vi "Main ver4.vi"(0 "PID On":bool) -> (5 "Total (V)":dbl[](array[slide]) scale=-8.0..8.0, 6 "Force (N)":T1(graph)={"M1 ref force"=19.690402476780186, "M2 ref force"=19.690402476780186, "M1 mes force"=5.466389475814116, "M2 mes force"=1.4423805363163493})   [LabVIEW 2021]
uses:
  <vilib>/Platform/TimedLoop/XDataNode/timing_clust.ctl
  <vilib>/Platform/TimedLoop/XDataNode/nitl_modes.ctl
  <vilib>/Platform/TimedLoop/XDataNode/wakeup.ctl
  <vilib>/Analysis/3filter.llb/Filter Passband Type.ctl
  <vilib>/Analysis/baseanly.llb/Real Dot Product.vi
  <vilib>/DAQmx/write.llb/DAQmx Write (Digital 1D Bool 1Chan 1Samp).vi
  <vilib>/DAQmx/write.llb/DAQmx Write (Analog 1D DBL NChan 1Samp).vi
  <vilib>/DAQmx/create/channels.llb/DAQmx Create Channel (DO-Digital Output).vi
  <vilib>/DAQmx/create/channels.llb/DAQmx Create Channel (AO-Voltage-Basic).vi
  <vilib>/DAQmx/create/channels.llb/DAQmx Create Channel (AI-Voltage-Basic).vi
  <vilib>/DAQmx/configure/timing.llb/DAQmx Timing (Sample Clock).vi
  <vilib>/addons/control/pid/pid.llb/PID (DBL).vi
  <vilib>/DAQmx/miscellaneous.llb/DAQmx Fill In Error Info.vi
  <vilib>/platform/TimedLoop/XDataNode/XDataNode.xnode
  <vilib>/addons/control/pid/NI_PID_pid.lvlib
  <vilib>/Platform/TimedLoop/XDataNode/XDNodeRunTimeDep.lvlib
  <vilib>/Analysis/NI_AALBase.lvlib
  <vilib>/ptbypt/NI_PtbyPt.lvlib
panel:
  out "Force (N) 2":T1(graph)={"M1 ref force"=19.938080495356036, "M2 ref force"=19.938080495356036, "M1 mes force"=7.2507342741854055, "M2 mes force"=-127.25356072908707}
  in  "Gains 2":T2(array[cluster])=[{"proportional gain (Kc)"=0.17, "integral time (Ti, min)"=0.0, "derivative time (Td, min)"=0.0}, {"proportional gain (Kc)"=0.17, "integral time (Ti, min)"=0.0, "derivative time (Td, min)"=0.0}] {"derivative time (Td, min)" format="%.3f"; "integral time (Ti, min)" format="%.3f"; "proportional gain (Kc)" format="%.3f"}
  in  "Torque":dbl[](array[numeric])=[0.15, 0.15]
  out "Speed":dbl[](array[numeric])
  in  "Record?":bool
  out "XY Graph":cluster{dbl[], dbl[]}[](graph)=[{[0.0, 26.31578947368421, 52.63157894736842, 78.94736842105263, 105.26315789473684, 131.57894736842104, 157.89473684210526, 184.21052631578945, 210.52631578947367, 236.8421052631579, 263.1578947368421, 289.4736842105263, 315.7894736842105, 342.10526315789474, 368.4210526315789, 394.7368421052631, 421.05263157894734, 447.36842105263156, 473.6842105263158, 499.99999999999994], [0.0, 0.0, 0.0, 0.0, 0.0, 0.0, 0.0, 0.0, 0.0, 0.0, 0.0, 0.0, 0.0, 0.0, 0.0, 0.0, 0.0, 0.0, 0.0, 0.0]}, {[0.0, 26.31578947368421, 52.63157894736842, 78.94736842105263, 105.26315789473684, 131.57894736842104, 157.89473684210526, 184.21052631578945, 210.52631578947367, 236.8421052631579, 263.1578947368421, 289.4736842105263, 315.7894736842105, 342.10526315789474, 368.4210526315789, 394.7368421052631, 421.05263157894734, 447.36842105263156, 473.6842105263158, 499.99999999999994], [0.0, 0.0, 0.0, 0.0, 0.0, 0.0, 0.0, 0.0, 0.0, 0.0, 0.0, 0.0, 0.0, 0.0, 0.0, 0.0, 0.0, 0.0, 0.0, 0.0]}, {[0.0, 26.31578947368421, 52.63157894736842, 78.94736842105263, 105.26315789473684, 131.57894736842104, 157.89473684210526, 184.21052631578945, 210.52631578947367, 236.8421052631579, 263.1578947368421, 289.4736842105263, 315.7894736842105, 342.10526315789474, 368.4210526315789, 394.7368421052631, 421.05263157894734, 447.36842105263156, 473.6842105263158, 499.99999999999994], [0.0, 0.0, 0.0, 0.0, 0.0, 0.0, 0.0, 0.0, 0.0, 0.0, 0.0, 0.0, 0.0, 0.0, 0.0, 0.0, 0.0, 0.0, 0.0, 0.0]}, {[0.0, 26.31578947368421, 52.63157894736842, 78.94736842105263, 105.26315789473684, 131.57894736842104, 157.89473684210526, 184.21052631578945, 210.52631578947367, 236.8421052631579, 263.1578947368421, 289.4736842105263, 315.7894736842105, 342.10526315789474, 368.4210526315789, 394.7368421052631, 421.05263157894734, 447.36842105263156, 473.6842105263158, 499.99999999999994], [0.0, 0.0, 0.0, 0.0, 0.0, 0.0, 0.0, 0.0, 0.0, 0.0, 0.0, 0.0, 0.0, 0.0, 0.0, 0.0, 0.0, 0.0, 0.0, 0.0]}]
  out "Period":i64=2
  out "Finished Late? [i-1]":bool
  in  "Tab Control 2":enum32{"Initialize", "RBF"}(tab)
  in  "Encoder":bool
  in  "Loadcell":bool
  in  "Set Tension":dbl=10.0
  in  "x":cluster{"Number":i32, "x_0":dbl, "x_f":dbl}={"Number"=20, "x_0"=0.0, "x_f"=500.0}
  out "Output":dbl(slide)=nan scale=0.0..10.0
  out "Weights":dbl[](array[numeric])
  in  "RBF 2":cluster{"STD":dbl, "Number":i32}={"STD"=150.0, "Number"=3}
  in  "Traj Start":i32(knob)=1 scale=0.0..2.0
  in  "Tab Control":enum32{"Page 1", "Position"}(tab)=enum."Position"
  out "RPM":cluster{"Position":dbl, "ref_x (mm)":dbl}(graph)
  out "Position (mm)":cluster{"Position":dbl, "ref_x (mm)":dbl}(graph)={"Position"=0.0, "ref_x (mm)"=500.0}
  in  "RBF":bool
  in  "Set Point":dbl(slide)=19.938080495356036 scale=0.0..40.0
  in  "stop":bool
  in  "Tab Control 3":enum32{"Current", "PID On", "Position"}(tab)=enum."PID On"
  in  "Gains":T2(array[cluster])=[{"proportional gain (Kc)"=0.17, "integral time (Ti, min)"=0.0, "derivative time (Td, min)"=0.0}, {"proportional gain (Kc)"=0.17, "integral time (Ti, min)"=0.0, "derivative time (Td, min)"=0.0}] {"derivative time (Td, min)" format="%.3f"; "integral time (Ti, min)" format="%.3f"; "proportional gain (Kc)" format="%.3f"}
  out "PID (V)":dbl[](array[slide])=[2.9907120743034055, 2.9907120743034055] scale=-8.0..10.0
  in  "Motor Enable":bool[](array[boolean])=[FALSE, FALSE]
  in  "Damping":dbl[](array[numeric])=[0.0, 0.0]
  in  "PID gains":T3={"proportional gain (Kc)"=0.1, "integral time (Ti, min)"=0.0, "derivative time (Td, min)"=0.0} {"derivative time (Td, min)" format="%.3f"; "integral time (Ti, min)" format="%.3f"; "proportional gain (Kc)" format="%.3f"}
  in  "Pos Control":bool
  out "output":dbl(slide)=50.0 scale=-40.0..40.0
  # "TRAJECTORY"
  # "FORCE"
  # "INITIALIZE"
  # "TUNE"
  # "MONITOR"
  # "DEVEL"
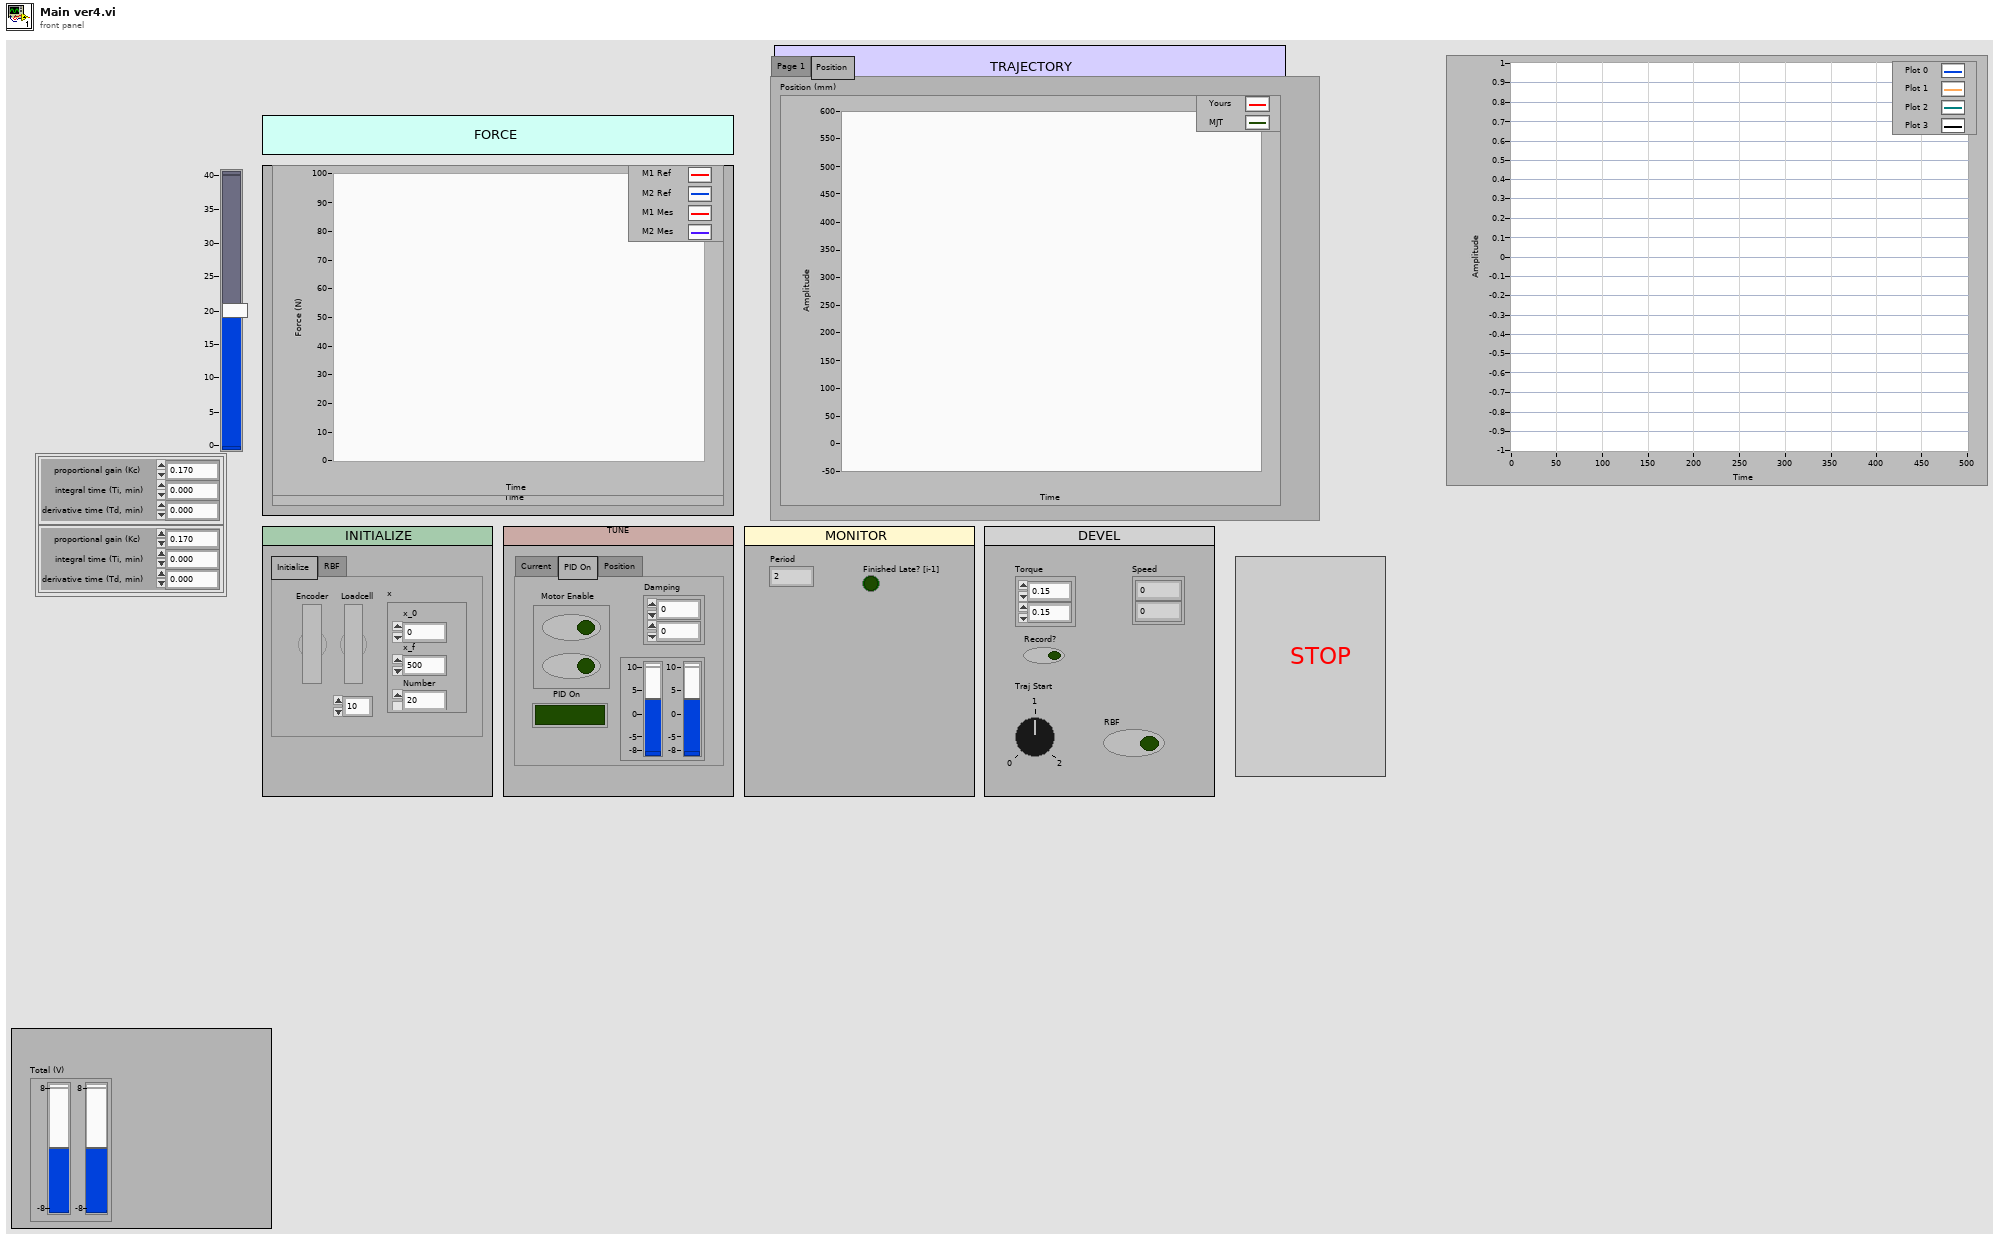
[diagram p1: front panel]
types:
  T1 = cluster{"M1 ref force":dbl, "M2 ref force":dbl, "M1 mes force":dbl, "M2 mes force":dbl}
  T2 = cluster{"proportional gain (Kc)":dbl, "integral time (Ti, min)":dbl, "derivative time (Td, min)":dbl}[]
  T3 = cluster{"proportional gain (Kc)":dbl, "integral time (Ti, min)":dbl, "derivative time (Td, min)":dbl}
  T4 = enum16{"open", "open or create", "create or replace", "create", "open (read-only)"}
  T5 = typedef "XDNodeRunTimeDep.lvlib/timing_clust.ctl" = cluster{"Expected End [f-1]":u64, "Actual End [f-1]":u64, "Finished Late? [f-1]":bool, "Expected End [i-1]":u64, "Actual End [i-1]":u64, "Finished Late? [i-1]":bool, "Expected Start [i]":u64, "Actual Start [i]":u64, "Expected Start [f]":u64, "Actual Start [f]":u64, "Source Name":string, "Structure Name":string, "Period":i64, "Deadline":i64, "Offset":i64, "Start":i64, "Priority":i32, "Timeout":i32, "Mode":T6, "Wakeup Reason":T7, "Error":errorcluster, "Source Type":string, "Secondary Source Type":string, "Global End Time":u64, "Global Start Time":u64, "Frame Duration":u64, "Iteration Duration":u64, "Assigned CPU":i32, "I/O Scan Engine Mode":u32}
  T6 = typedef "XDNodeRunTimeDep.lvlib/nitl_modes.ctl" = enum32{"No Change", "Process missed periods, maintain original phase", "Discard missed periods, maintain original phase", "Process missed periods, ignore original phase", "Discard missed periods, ignore original phase"}
  T7 = typedef "XDNodeRunTimeDep.lvlib/wakeup.ctl" = enum32{"Normal", "Aborted", "Asynchronous wakeup", "Timing source error", "Timed loop error", "Timeout"}
  T8 = typedef "NI_AALBase.lvlib/Filter Passband Type.ctl" = enum32{"Lowpass", "Highpass", "Bandpass", "Bandstop"}
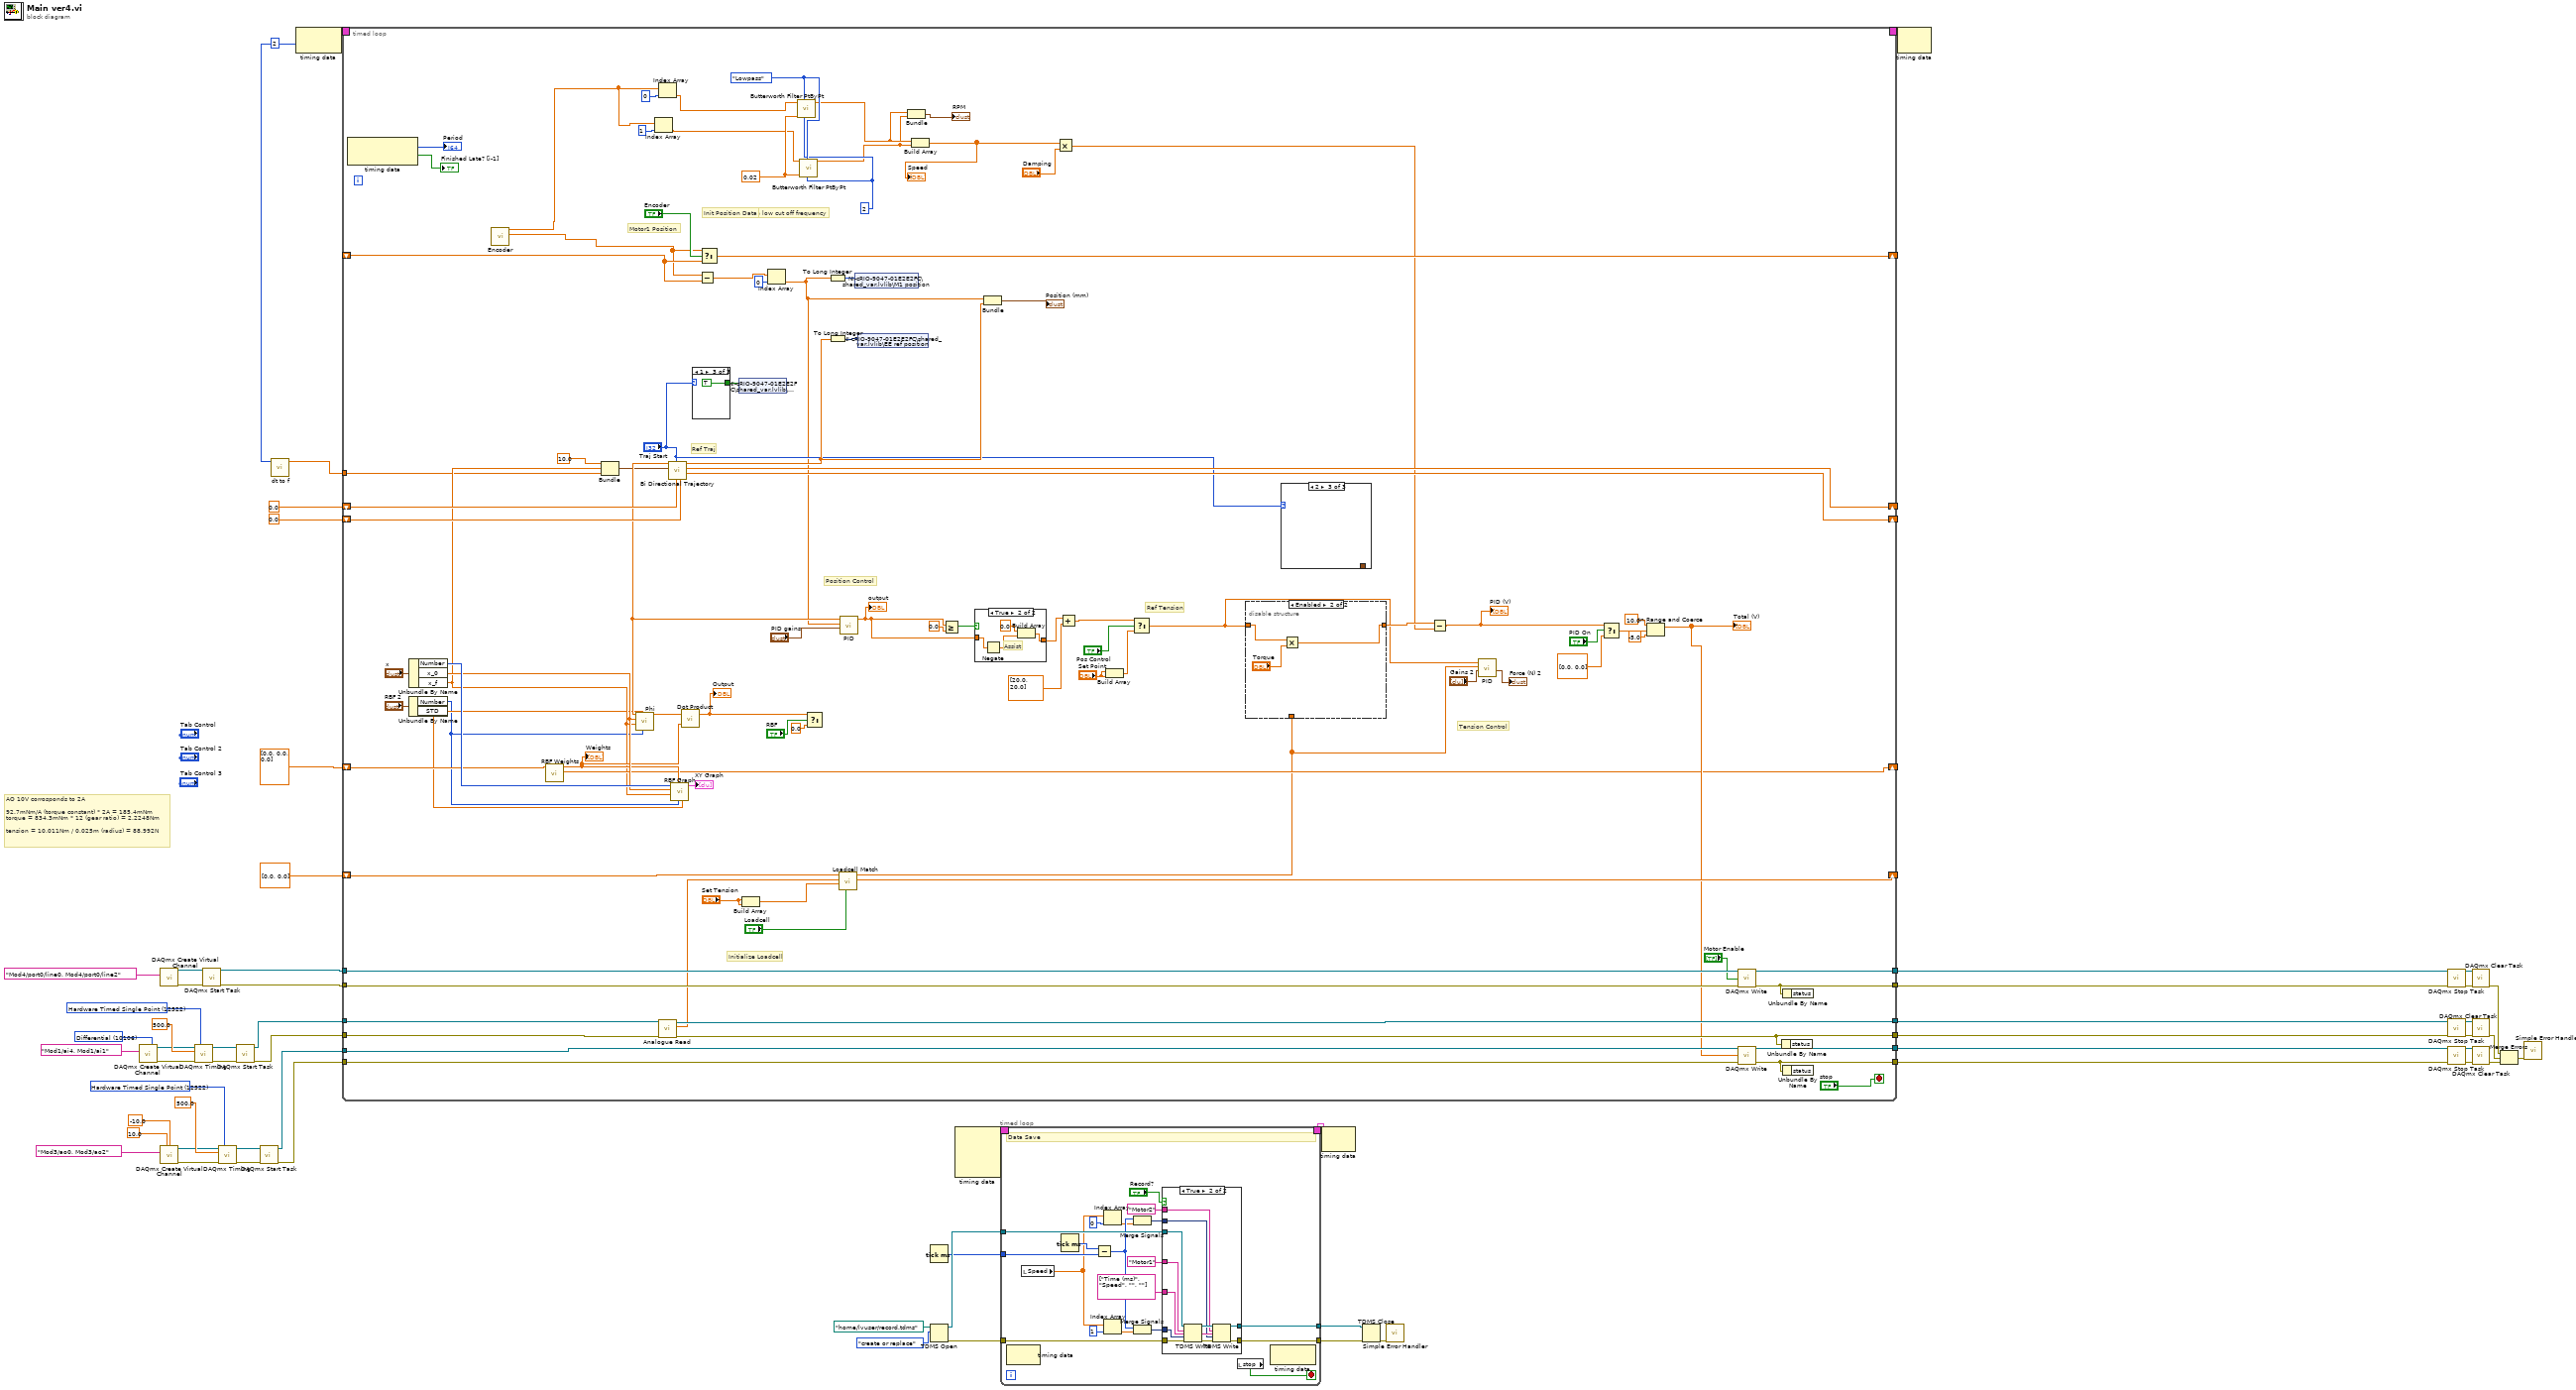
[diagram p0: block diagram]
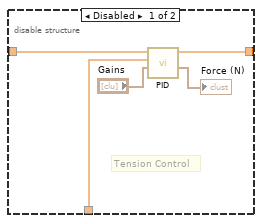
[diagram p3: hidden frame]
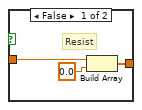
[diagram p4: hidden frame]
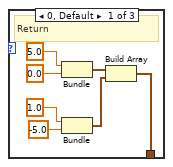
[diagram p5: hidden frame]
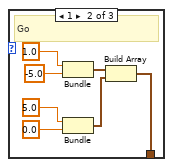
[diagram p6: hidden frame]
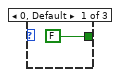
[diagram p7: hidden frame]
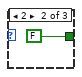
[diagram p8: hidden frame]
diagram:
  w15 = 12522 items=["Finite Samples"=10178, "Continuous Samples"=10123, "Hardware Timed Single Point"=12522] ("sample mode")
  w18 = 12522 items=["Finite Samples"=10178, "Continuous Samples"=10123, "Hardware Timed Single Point"=12522] ("sample mode")
  w25 = i64 2 ("Period")
  w32 = 10106 items=["Default"=-1, "RSE"=10083, "NRSE"=10078, "Differential"=10106, "Pseudodifferential"=12529] ("input terminal configuration")
  # "AO 10V corrosponds to 2A\n\n92.7mNm/A (torque constant) * 2A = 185.4mNm\ntorque = 834.3mNm * 12 (gear ratio) = 2.2248Nm\n\ntension = 10.011Nm / 0.025m (radius) = 88.992N"
  n1 = call-poly <vilib>:"DAQmx Create Virtual Channel.vi"("input terminal configuration"=w32, "physical channels"=tag "Mod1/ai4, Mod1/ai1") -> ("task out"=w22:refnum<k21>, "error out"=w21:errorcluster)  [unwired: 12 in]
  n2 = call-poly <vilib>:"DAQmx Create Virtual Channel.vi"("lines"=tag "Mod4/port0/line0, Mod4/port0/line2") -> ("task out"=w17:refnum<k21>, "error out"=w54:errorcluster)  [unwired: 13 in]
  n3 = call-poly <vilib>:"DAQmx Create Virtual Channel.vi"("maximum value"=10.0 ("AO max"), "minimum value"=-10.0 ("AO min"), "physical channels"=tag "Mod3/ao0, Mod3/ao2" ("Physical Channel(s)")) -> ("task out"=w14:refnum<k21>, "error out"=w12:errorcluster)  [unwired: 11 in]
  n4 = call-poly <vilib>:"DAQmx Timing.vi"("task/channels in"=w22, "sample mode"=w18, "rate"=500.0, "error in"=w21) -> ("task out"=w19:refnum<k21>, "error out"=w20:errorcluster)  [unwired: 10 in]
  n5 = call <vilib>:"DAQmx Start Task.vi"("task/channels in"=w17, "error in"=w54) -> ("task out"=w52:refnum<k21>, "error out"=w51:errorcluster)  [unwired: 12 in]
  n6 = call-poly <vilib>:"DAQmx Timing.vi"("task/channels in"=w14, "sample mode"=w15, "rate"=500.0, "error in"=w12) -> ("task out"=w13:refnum<k21>, "error out"=w11:errorcluster)  [unwired: 10 in]
  n7 = call <vilib>:"DAQmx Start Task.vi"("task/channels in"=w19, "error in"=w20) -> ("task out"=w45:refnum<k21>, "error out"=w44:errorcluster)  [unwired: 12 in]
  n8 = call <vilib>:"DAQmx Start Task.vi"("task/channels in"=w13, "error in"=w11) -> ("task out"=w56:refnum<k21>, "error out"=w55:errorcluster)  [unwired: 12 in]
  n9 = call "dt to f.vi"("Period"=w25) -> ("Frequency"=w24:dbl)  [unwired: 10 in]
  n10 = node-c288(w25) -> (w28:T5)
  n11 = timed-loop {
    tunnel: [w153] -> w60
    tunnel: [w152] -> w59
    tunnel: [w139] -> w58
    tunnel: [w144] -> w57
    tunnel: w45 -> [w150]
    tunnel: w44 -> [w149]
    tunnel: w56 -> [w138]
    tunnel: w55 -> [w151]
    tunnel: w52 -> [w148]
    tunnel: w51 -> [w147]
    tunnel: [w146] -> w48
    tunnel: [w145] -> w47
    shift-right: [w142] -> _
    shift-left: 0.0 ("total time") -> [w143]
    shift-right: [w141] -> _
    shift-left: _ -> [w140]
    shift-right: [w136] -> _
    shift-left: dbl[] [0.0, 0.0] ("measured force") -> [w137]
    shift-right: [w134] -> _
    shift-left: 0.0 ("total time") -> [w135]
    timing: w28 -> [_]
    timing-out: [_] -> w27
    shift-right: [w101] -> _
    shift-left: dbl[] [0.0, 0.0, 0.0] ("Array of Double") -> [w102]
    tunnel: w24 -> [w93]
    stop <- "stop" stop-if-true
    w83 = 2 ("order")
    w85 = 0.02 ("low cutoff freq: fl")
    w84 = Filter_Passband_Type."Lowpass" ("filter type")
    # "Tension Control"
    # "change low cut off frequency"
    # "Initialize Loadcell"
    # "Ref Tension"
    # "Position Control"
    # "Ref Traj"
    # "Init Position Data"
    # "Motor1 Position"
    n12 = node-c288() -> (→"Period":i64, →"Finished Late? [i-1]":bool)  [unwired: 1 in]
    n13 = Unbundle By Name("RBF 2") -> ("Number"=w89:i32, "STD"=w90:dbl)
    n14 = Unbundle By Name("x") -> ("Number"=w111:i32, "x_0"=w108:dbl, "x_f"=w94:dbl)
    n15 = call "Encoder.vi"() -> ("Mes Pos (mm)"=w72:dbl[], "RPM"=w80:dbl[])  [unwired: 10 in]
    n16 = call "RBF Weights.vi"("Array of Double in"=w102) -> ("Array of Double out"=w101:dbl[], "Array of Double 3"=w103:dbl[])  [unwired: 9 in]
    "Weights" <- w103
    n17 = Bundle("y"=10.0, "x_f"=w94, "Frequency"=w93) -> (w92:cluster{"y":dbl, "x_f":dbl, "Frequency":dbl})  [unwired: 1 in]
    n18 = Index Array(array=w80, index=1) -> (element=w78:dbl)
    n19 = Index Array(array=w80, index=0) -> (element=w79:dbl)
    n20 = call "Analogue Read.vi"("error in"=w149, "task/channels in"=w150) -> ("error out"=w144:errorcluster, "measured force"=w120:dbl[], "task out"=w139:refnum<k21>)  [unwired: 6 in, 1 out]
    n21 = call "Bi Directional Trajectory.vi"("Return Time"=w135, "Go Time"=w143, "Traj Start"="Traj Start", "Trajectory Settings"=w92) -> ("Return Next Time"=w134:dbl, "Go Next Time"=w142:dbl, "Output (mm)"=w107:dbl)  [unwired: 5 in]
    n22 = call "Phi.vi"("Number"=w89, "STD"=w90, "x_f"=w94, "x_0"=w108, "Output (mm)"=w107) -> ("Array"=w106:dbl[])  [unwired: 6 in]
    n23 = call "RBF Graph.vi"("STD"=w90, "Number"=w89, "Array of Double 3"=w103, "x_f"=w94, "x_0"=w108, "Number 2"=w111) -> ("Array"=→"XY Graph":cluster{dbl[], dbl[]}[])  [unwired: 5 in]
    n24 = call-poly <vilib>:"Dot Product.vi"("Y Vector"=w103, "X Vector"=w106) -> ("X * Y"=w100:dbl)  [unwired: 1 out]
    "Output" <- w100
    n25 = case shown="1" "Traj Start" {
      tunnel: [FALSE FALSE TRUE] -> w104
      frame 0, Default {
      }
      frame 2 {
      }
      frame 1 {
      }
    }
    n26 = Subtract(x=w72, y=w140) -> (x-y=w71:dbl[])
    n27 = Select(t=w72, s="Encoder", f=w140) -> (s? t:f=w141:dbl[])
    n28 = shared-variable "NI-cRIO-9047-01E2E2FC\\shared_var.lvlib\\Trigger"(w104) -> ()  [unwired: 1 in, 1 out]
    n29 = Build Array("Set Tension", "Set Tension") -> (w118:dbl[])
    n30 = Index Array(array=w71, index=0) -> (element=w70:dbl)
    n31 = call <vilib>:"Butterworth Filter PtByPt.vi"("order"=w83, "filter type"=w84, "low cutoff freq: fl"=w85, "x"=w79) -> ("Filtered x"=w68:dbl)  [unwired: 5 in, 1 out]
    n32 = call <vilib>:"Butterworth Filter PtByPt.vi"("order"=w83, "filter type"=w84, "low cutoff freq: fl"=w85, "x"=w78) -> ("Filtered x"=w67:dbl)  [unwired: 5 in, 1 out]
    n33 = Select(t=w100, s="RBF", f=0.0) -> ()  [unwired: 1 out]
    n34 = To Long Integer(number=w70) -> (32bit integer=w114:i32)
    n35 = To Long Integer(number=w107) -> (32bit integer=w115:i32)
    n36 = call "Loadcell Match.vi"("Initialize"="Loadcell", "Set Tension"=w118, "Mes Tension"=w120, "Next Tension Error"=w137) -> ("Tension Error"=w136:dbl[], "Filtered Tension"=w61:dbl[])  [unwired: 6 in]
    n37 = call-poly <vilib>:"PID.vi"("PID gains"="PID gains", "process variable"=w70, "setpoint"=w107) -> ("output"=w86:dbl)  [unwired: 7 in, 1 out]
    "output" <- w86
    n38 = shared-variable "NI-cRIO-9047-01E2E2FC\\shared_var.lvlib\\M1 position"(w114) -> ()  [unwired: 1 in, 1 out]
    n39 = shared-variable "NI-cRIO-9047-01E2E2FC\\shared_var.lvlib\\EE ref position"(w115) -> ()  [unwired: 1 in, 1 out]
    n40 = Bundle("Filtered x"=w68, "Filtered x"=w67) -> (→"RPM":cluster{"Filtered x":dbl, "Filtered x":dbl})  [unwired: 1 in]
    n41 = Build Array(w68, w67) -> (w65:dbl[])
    "Speed" <- w65
    n42 = Greater Or Equal?(x=w86, y=0.0) -> (x >= y?=w99:bool)
    n43 = case shown="True" w99 {
      tunnel: w86 -> [w165 w169]
      tunnel: [w167 w171] -> w96
      frame False {
        # "Resist"
        n44 = Build Array(w165, 0.0 ("element")) -> (w167:dbl[])
      }
      frame True {
        # "Assist"
        n45 = Negate(x=w169) -> (-x=w168:dbl)
        n46 = Build Array(0.0 ("element"), w168) -> (w171:dbl[])
      }
    }
    n47 = Bundle("Position"=w70, "Output (mm)"=w107) -> (→"Position (mm)":cluster{"Position":dbl, "Output (mm)":dbl})  [unwired: 1 in]
    n48 = Multiply(x=w65, y="Damping") -> (x*y=w69:dbl[])
    n49 = Add(x=w96, y=dbl[] [20.0, 20.0] ("x")) -> (x+y=w95:dbl[])
    n50 = Build Array("Set Point", "Set Point") -> (w128:dbl[])
    n51 = Select(t=w95, s="Pos Control", f=w128) -> (s? t:f=w62:dbl[])
    n52 = disable-structure shown="Enabled" {
      disable-tunnel: w61 -> [w157 _]
      disable-tunnel: [w155 w160] -> w76
      disable-tunnel: w62 -> [w154 w161]
      frame Disabled {
        # "Tension Control"
        n53 = call <vilib>:"PID.vi"("PID gains"="Gains", "mes force"=w157, "ref force"=w154) -> ("output cluster"=→"Force (N)":T1, "PID output"=w155:dbl[])  [unwired: 7 in]
      }
      frame Enabled {
        n54 = Multiply(x=w161, y="Torque") -> (x*y=w160:dbl[])
      }
    }
    n55 = case shown="2" "Traj Start" {
      tunnel: [w172 w179 _] -> _
      frame 0, Default {
        # "Return"
        n56 = Bundle(5.0, 0.0) -> (w178:cluster{dbl, dbl})  [unwired: 1 in]
        n57 = Bundle(1.0, -5.0) -> (w177:cluster{dbl, dbl})  [unwired: 1 in]
        n58 = Build Array(w178, w177) -> (w172:cluster{dbl, dbl}[])
      }
      frame 1 {
        # "Go"
        n59 = Bundle(1.0, -5.0) -> (w180:cluster{dbl, dbl})  [unwired: 1 in]
        n60 = Bundle(5.0, 0.0) -> (w181:cluster{dbl, dbl})  [unwired: 1 in]
        n61 = Build Array(w180, w181) -> (w179:cluster{dbl, dbl}[])
      }
      frame 2 {
      }
    }
    n62 = Subtract(x=w76, y=w69) -> (x-y=w75:dbl[])
    "PID (V)" <- w75
    n63 = call <vilib>:"PID.vi"("PID gains"="Gains 2", "mes force"=w61, "ref force"=w62) -> ("output cluster"=→"Force (N) 2":T1)  [unwired: 7 in, 1 out]
    n64 = Select(t=w75, s="PID On", f=dbl[] [0.0, 0.0]) -> (s? t:f=w130:dbl[])
    n65 = In Range and Coerce(upper limit=10.0, x=w130, lower limit=-5.0) -> (coerced(x)=w116:dbl[])  [unwired: 1 out]
    "Total (V)" <- w116
    n66 = call-poly <vilib>:"DAQmx Write.vi"("task/channels in"=w148, "data"="Motor Enable", "error in"=w147) -> ("task out"=w146:refnum<k21>, "error out"=w145:errorcluster)  [unwired: 10 in, 1 out]
    n67 = call-poly <vilib>:"DAQmx Write.vi"("task/channels in"=w138, "data"=w116, "error in"=w151) -> ("task out"=w153:refnum<k21>, "error out"=w152:errorcluster)  [unwired: 10 in, 1 out]
    n68 = Unbundle By Name(w144) -> ()  [unwired: 1 out]
    n69 = Unbundle By Name(w145) -> ()  [unwired: 1 out]
    n70 = Unbundle By Name(w152) -> ()  [unwired: 1 out]
  }
  n71 = Tick Count (ms)() -> (millisecond timer value=w3:u32)
  n72 = TDMS Open(10:T4."create or replace" ("operation (0:open)"), 11:path "/home/lvuser/record.tdms" ("file path")) -> (0:w6:errorcluster, 3:w10:refnum<k34>)  [unwired: 5 in]
  n73 = node-c288() -> (w2:T5)  [unwired: 4 in]
  n74 = timed-loop {
    tunnel: w10 -> [w208]
    tunnel: [w204] -> w9
    tunnel: [w205] -> w7
    tunnel: w6 -> [w207]
    tunnel: w3 -> [w198]
    timing: w2 -> [_]
    timing-out: [_] -> w1
    stop <- w196 stop-if-true
    # "Data Save"
    n75 = node-c288() -> ()  [unwired: 1 in, 1 out]
    n76 = local read "Speed"() -> (w190:dbl[])
    n77 = Tick Count (ms)() -> (millisecond timer value=w199:u32)
    n78 = Subtract(x=w199, y=w198) -> (x-y=w197:u32)
    n79 = Index Array(array=w190, index=0) -> (element=w192:dbl)
    n80 = Index Array(array=w190, index=1) -> (element=w191:dbl)
    n81 = Merge Signals(w197, w192) -> (w200:dynamicdata)
    n82 = Merge Signals(w197, w191) -> (w201:dynamicdata)
    n83 = case shown="True" "Record?" {
      tunnel: w208 -> [w209 w222]
      tunnel: w207 -> [w210 w221]
      tunnel: "Motor1" ("group name in (Untitled)") -> [_ w220]
      tunnel: [w210 w218] -> w205
      tunnel: [w209 w216] -> w204
      tunnel: "Motor2" ("group name in (Untitled)") -> [_ w215]
      tunnel: string[] ["Time (ms)", "Speed", "", ""] ("channel name(s) in (Untitled)") -> [_ w214]
      tunnel: w201 -> [_ w212]
      tunnel: w200 -> [_ w211]
      frame False {
      }
      frame True {
        n84 = TDMS Write(0:w222, 5:w220, 7:w214, 9:w212, 11:w221) -> (4:w217:refnum<k34>, 8:w213:string[], 15:w219:errorcluster)  [unwired: 1 in, 1 out]
        n85 = TDMS Write(0:w217, 5:w215, 7:w213, 9:w211, 11:w219) -> (4:w216:refnum<k34>, 15:w218:errorcluster)  [unwired: 1 in, 2 out]
      }
    }
    n86 = local read "stop"() -> (w196:bool)
    n87 = node-c288() -> ()  [unwired: 1 in, 1 out]
  }
  n88 = node-c288(w1) -> ()  [unwired: 1 out]
  n89 = TDMS Close(8:w7, 11:w9) -> (0:w8:errorcluster)  [unwired: 1 out]
  n90 = call <vilib>:"Simple Error Handler.vi"("error in (no error)"=w8) -> ()  [unwired: 4 in, 5 out]
  n91 = node-c288(w27) -> ()  [unwired: 1 out]
  n92 = call <vilib>:"DAQmx Stop Task.vi"("task/channels in"=w48, "error in"=w47) -> ("task out"=w50:refnum<k21>, "error out"=w49:errorcluster)  [unwired: 12 in]
  n93 = call <vilib>:"DAQmx Stop Task.vi"("task/channels in"=w58, "error in"=w57) -> ("task out"=w38:refnum<k21>, "error out"=w37:errorcluster)  [unwired: 12 in]
  n94 = call <vilib>:"DAQmx Stop Task.vi"("task/channels in"=w60, "error in"=w59) -> ("task out"=w40:refnum<k21>, "error out"=w39:errorcluster)  [unwired: 12 in]
  n95 = call <vilib>:"DAQmx Clear Task.vi"("task in"=w50, "error in"=w49) -> ("error out"=w33:errorcluster)  [unwired: 13 in]
  n96 = call <vilib>:"DAQmx Clear Task.vi"("task in"=w38, "error in"=w37) -> ("error out"=w34:errorcluster)  [unwired: 13 in]
  n97 = call <vilib>:"DAQmx Clear Task.vi"("task in"=w40, "error in"=w39) -> ("error out"=w35:errorcluster)  [unwired: 13 in]
  n98 = Merge Errors(w33, w34, w35) -> (w36:errorcluster)
  n99 = call <vilib>:"Simple Error Handler.vi"("error in (no error)"=w36) -> ()  [unwired: 4 in, 5 out]
